vi "DSF.Engine.Plugin.Tx.Inline.Start.vi"(8 "error in (no error)":errorcluster, 11 "Plugin in":refnum<class "DSF.Engine.Plugin.lvclass">) -> (0 "error out":errorcluster, 3 "Plugin out":refnum<class "DSF.Engine.Plugin.lvclass">)   [LabVIEW 2017, in "DSF.Engine.lvlib" / "DSF.Engine.Plugin.lvclass"]
uses:
  DSF.Engine.Plugin.lvclass
  DSF.Engine.Plugin.lvclass/DSF.Engine.Plugin.ctl
  Interface/DSF.Engine.Interface.Transceiver.Command.ctl
  Transfer/DSF.Engine.Transfer Group.lvclass/DSF.Engine.Transfer Group.ctl
  Timing/DSF.Engine.Timing.lvclass/DSF.Engine.Timing.ctl
  Timing/DSF.Engine.Timing.Iteration.Increment.vi
  Interface/DSF.Engine.Interface.Transceiver.lvclass
  Transfer/DSF.Engine.Transfer Group.lvclass
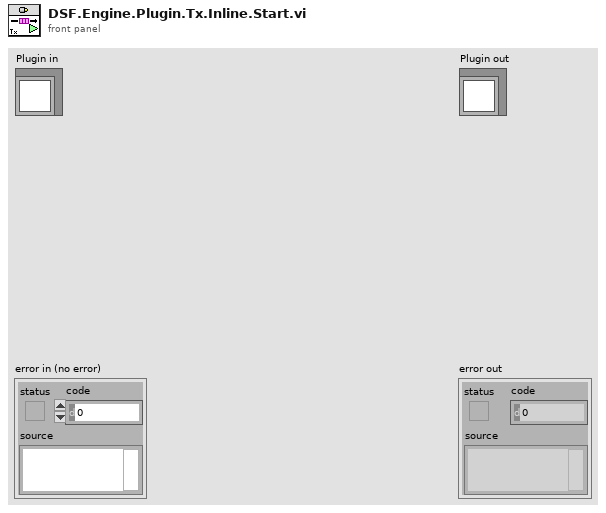
[diagram p1: front panel]
types:
  T1 = typedef "DSF.Engine.lvlib/DSF.Engine.Interface.Transceiver.lvclass/DSF.Engine.Interface.Transceiver.Command.ctl" = enum8{"Set Base Pointer", "Rx", "Tx", "Shutdown"}
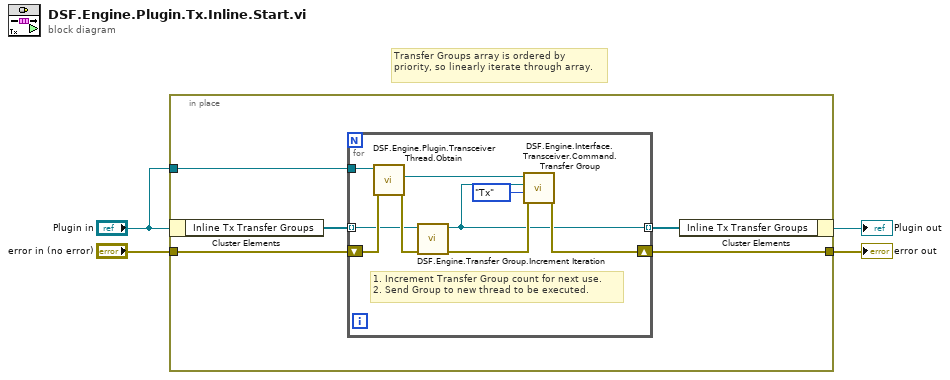
[diagram p0: block diagram]
diagram:
  # "Transfer Groups array is ordered by priority, so linearly iterate through array."
  n1 = in-place {
    in-place-border: "error in (no error)" -> [w9]
    in-place-border: [w8] -> w3
    in-place-border: "Plugin in" -> [w5]
    n2 = in-place-cluster #1("Plugin in") -> ("Inline Tx Transfer Groups"=w7:refnum<class "DSF.Engine.Transfer Group.lvclass">[])
    n3 = for {
      tunnel: w7 -> [w14] mode=indexing
      shift-right: [w11] -> w8
      shift-left: w9 -> [w16]
      tunnel: [w10] -> w6 mode=indexing
      tunnel: w5 -> [w17]
      # "1. Increment Transfer Group count for next use.\n2. Send Group to new thread to be executed."
      n4 = call "DSF.Engine.Plugin.Transceiver Thread.Obtain.vi"("error in (no error)"=w16, "Plugin in"=w17) -> ("error out"=w15:errorcluster, "Transceiver Thread"=w18:refnum<class "DSF.Engine.Interface.Transceiver.lvclass">)  [unwired: 7 in, 1 out]
      n5 = call "DSF.Engine.Transfer Group.Increment Iteration.vi"("error in (no error)"=w15, "Transfer Group in"=w14) -> ("error out"=w12:errorcluster, "Transfer Group out"=w10:refnum<class "DSF.Engine.Transfer Group.lvclass">)  [unwired: 8 in]
      n6 = call "DSF.Engine.Interface.Transceiver.Command.Transfer Group.vi"("error in (no error)"=w12, "Command"=DSF.Engine.Interface.Transceiver.Command."Tx", "Transfer Group"=w10, "Transceiver Interface in"=w18) -> ("error out"=w11:errorcluster)  [unwired: 6 in, 1 out]
    }
    n7 = in-place-cluster #1("Inline Tx Transfer Groups"=w6) -> (→"Plugin out":refnum<class "DSF.Engine.Plugin.lvclass">)
  }
  "error out" <- w3
